vi "LoadFrontEnd.vi"(8 "error in (no error)":errorcluster, 11 "FE_Name":string) -> (0 "error out":errorcluster, 3 "TestSetDef":T1={"General"={"ID"=0, "Model"="", "Dual Port?"=FALSE, "Options"="", "Options"={"E"=FALSE, "K"=FALSE, "H"=FALSE, "W"=FALSE, "F"=FALSE}, "Cal File"=path ""}, "Receiver"={"Fstart, MHz"=0.0, "Fstop MHz"=0.0, "Fstep MHz"=0.0, "IF, MHz"=0.0}, "RX Band"={"Fstart, MHz"=0.0, "Fstop MHz"=0.0}, "TX 1"={"Fstart, MHz"=0.0, "Fstop MHz"=0.0, "Pmax, dBm"=0.0, "Pstep, dB"=0.0}, "TX 2"={"Fstart, MHz"=0.0, "Fstop MHz"=0.0, "Pmax, dBm"=0.0, "Pstep, dB"=0.0}, "Low-side?"=TRUE})   [LabVIEW 2011]
uses:
  Test Set Definition.ctl
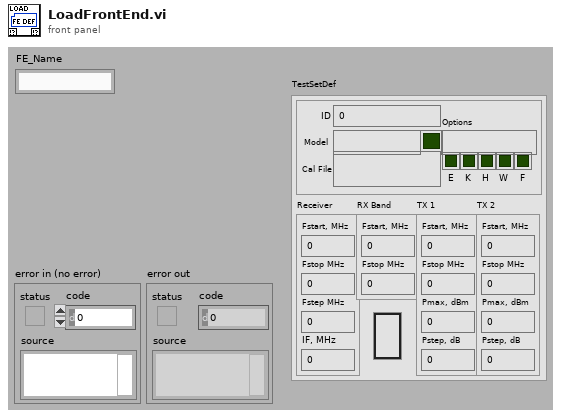
[diagram p1: front panel]
types:
  T1 = typedef "Test Set Definition.ctl" = cluster{"General":cluster{"ID":u32, "Model":string, "Dual Port?":bool, "Options":string, "Options":cluster{"E":bool, "K":bool, "H":bool, "W":bool, "F":bool}, "Cal File":path}, "Receiver":cluster{"Fstart, MHz":dbl, "Fstop MHz":dbl, "Fstep MHz":dbl, "IF, MHz":dbl}, "RX Band":cluster{"Fstart, MHz":dbl, "Fstop MHz":dbl}, "TX 1":cluster{"Fstart, MHz":dbl, "Fstop MHz":dbl, "Pmax, dBm":dbl, "Pstep, dB":dbl}, "TX 2":cluster{"Fstart, MHz":dbl, "Fstop MHz":dbl, "Pmax, dBm":dbl, "Pstep, dB":dbl}, "Low-side?":bool}
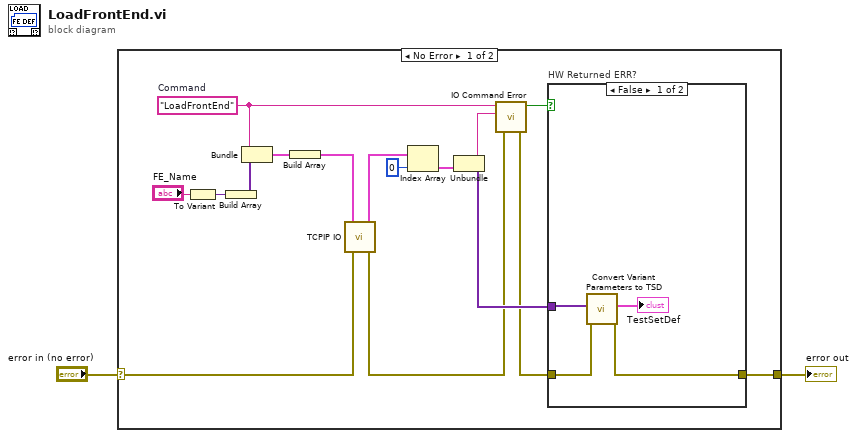
[diagram p0: block diagram]
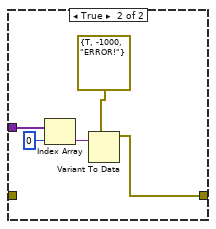
[diagram p2: hidden frame]
diagram:
  n1 = case shown="No Error" "error in (no error)" {
    selector: "error in (no error)" -> [w8 w28]
    tunnel: [w4 w28] -> w2
    frame No Error {
      w14 = "LoadFrontEnd"  # Command
      n2 = To Variant(anything="FE_Name") -> (Variant=w15:variant)
      n3 = Build Array(w15) -> (w18:variant[])
      n4 = Bundle("Command"=w14, w18) -> (w17:cluster{"Command":string, variant[]})  [unwired: 1 out]
      n5 = Build Array(w17) -> (w13:cluster{"Command":string, variant[]}[])
      n6 = call "TCPIP IO.vi"("error in (no error)"=w8, "Commands"=w13) -> ("error out"=w6:errorcluster, "Responses"=w12:cluster{string, variant[]}[])  [unwired: 1 in, 3 out]
      n7 = Index Array(array=w12, index=0) -> (element=w11:cluster{string, variant[]})
      n8 = Unbundle(w11) -> (w10:string, w7:variant[])
      n9 = call "IO Command Error.vi"("error in (no error)"=w6, "Command Returned (\"\")"=w10, "Command Sent (\"\")"=w14) -> ("error out"=w5:errorcluster, "HW ERR?"=w3:bool)  [unwired: 3 out]
      n10 = case "HW Returned ERR?" shown="False" w3 {
        tunnel: w7 -> [w20 w27]
        tunnel: w5 -> [w22 _]
        tunnel: [w21 w23] -> w4
        frame False {
          n11 = call "Convert Variant Parameters to TSD.vi"("error in"=w22, "Variant Parameter Array"=w20) -> ("error out"=w21:errorcluster, "TestSetDef"=→"TestSetDef":T1)  [unwired: 8 out]
        }
        frame True {
          n12 = Index Array(array=w27, index=0) -> (element=w25:variant)
          n13 = Variant To Data(type=errorcluster {"status"=TRUE, "code"=-1000, "source"="ERROR!"} ("error out"), Variant=w25) -> (data=w23:errorcluster)  [unwired: 1 in, 1 out]
        }
      }
    }
    frame Error {
    }
  }
  "error out" <- w2
